vi "_Drift_Compensator.vi"(7 "Device Number":T1, 9 "Zero Yaw":bool, 11 "Raw Yaw":dbl) -> (3 "comp yaw":dbl format="%#.1f")   [LabVIEW 2016]
uses:
  _TypeDefs/FRIC_navX_DeviceNumbersTypeDef.ctl
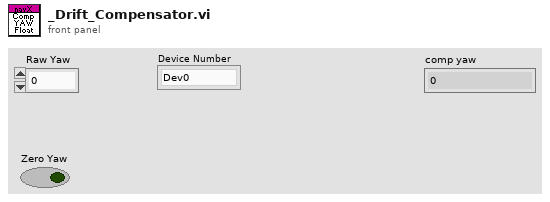
[diagram p1: front panel]
types:
  T1 = typedef "FRIC_navX_DeviceNumbersTypeDef.ctl" = enum16{"Dev0", "Dev1", "Dev2", "Dev3", "Dev4", "Dev5", "Dev6", "Dev7", "Dev8", "Dev9", "Dev10"}
  T2 = cluster{"current time":timestamp, "Error":dbl, "Drift error":dbl}
  T3 = cluster{"current time":timestamp, "Error":dbl, "Drift error":dbl}[]
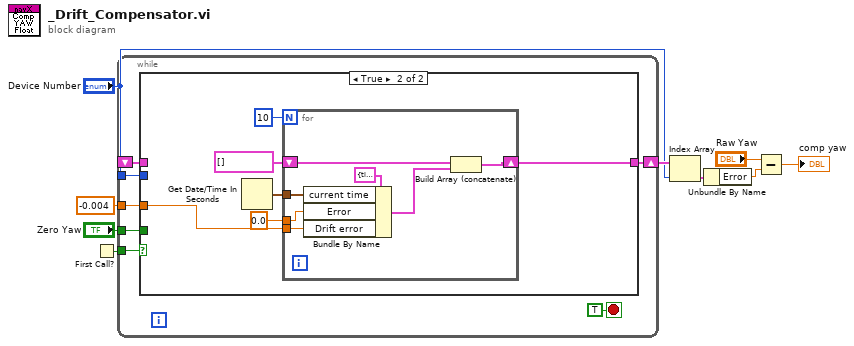
[diagram p0: block diagram]
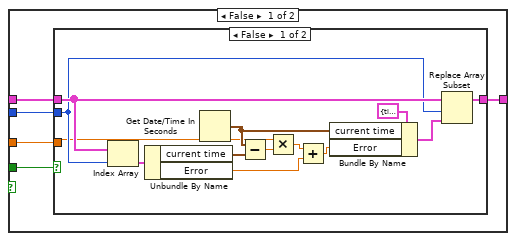
[diagram p2: hidden frame]
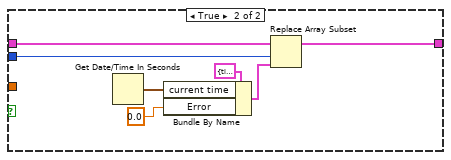
[diagram p3: hidden frame]
diagram:
  n1 = First Call?() -> (First Call?: T/F=w7:bool)
  n2 = while {
    shift-right: [w13] -> w5
    shift-left: _ -> [w12]
    tunnel: "Zero Yaw" -> [w15]
    tunnel: w7 -> [w14]
    tunnel: "Device Number" -> [w11]
    tunnel: -0.004 ("Dev0 Drift K/sec") -> [w10]
    stop <- TRUE stop-if-true
    n3 = case shown="True" w14 {
      tunnel: w15 -> [w21 _]
      tunnel: [w18 w45] -> w13
      tunnel: w12 -> [w20 _]
      tunnel: w11 -> [w19 _]
      tunnel: w10 -> [w17 w44]
      frame False {
        n4 = case shown="False" w21 {
          tunnel: w20 -> [w31 w41]
          tunnel: w19 -> [w29 w39]
          tunnel: [w30 w40] -> w18
          tunnel: w17 -> [w24 _]
          frame False {
            n5 = Index Array(array=w31, index=w29) -> (element=w33:T2)
            n6 = Unbundle By Name(w33) -> ("current time"=w32:timestamp, "Error"=w22:dbl)
            n7 = Get Date/Time In Seconds() -> (seconds since 1Jan1904=w25:timestamp)
            n8 = Subtract(x=w25, y=w32) -> (x-y=w34:dbl)
            n9 = Multiply(x=w24, y=w34) -> (x*y=w23:dbl)
            n10 = Add(x=w23, y=w22) -> (x+y=w26:dbl)
            n11 = Bundle By Name(cluster=T2 {"current time"=timestamp(0 s since 1904-01-01), "Error"=0.0, "Drift error"=0.0} ("new element/subarray"), "current time"=w25, "Error"=w26) -> (w27:T2)
            n12 = Replace Array Subset(array=w31, new element=w27, index=w29) -> (w30:T3)
          }
          frame True {
            n13 = Get Date/Time In Seconds() -> (seconds since 1Jan1904=w36:timestamp)
            n14 = Bundle By Name(cluster=T2 {"current time"=timestamp(0 s since 1904-01-01), "Error"=0.0, "Drift error"=0.0} ("new element/subarray"), "current time"=w36, "Error"=0.0) -> (w37:T2)
            n15 = Replace Array Subset(array=w41, new element=w37, index=w39) -> (w40:T3)
          }
        }
      }
      frame True {
        n16 = Get Date/Time In Seconds() -> (seconds since 1Jan1904=w47:timestamp)
        n17 = for {
          N: 10 ("dimension size") -> [_]
          tunnel: w47 -> [w53]
          shift-right: [w50] -> w45
          shift-left: T3 [] -> [w52]
          tunnel: w44 -> [w49]
          tunnel: 0.0 ("Error") -> [w48]
          n18 = Bundle By Name(cluster=T2 {"current time"=timestamp(0 s since 1904-01-01), "Error"=0.0, "Drift error"=-0.004447}, "current time"=w53, "Error"=w48, "Drift error"=w49) -> (w51:T2)
          n19 = Build Array (concatenate)(w52, w51) -> (w50:T3)
        }
      }
    }
  }
  n20 = Index Array(array=w5, index="Device Number") -> (element=w3:T2)
  n21 = Unbundle By Name(w3) -> ("Error"=w2:dbl)
  n22 = Subtract(x="Raw Yaw", y=w2) -> (x-y=→"comp yaw":dbl)
